vi "comm serial port list.vi"(8 "error in (no error)":errorcluster) -> (0 "error out":errorcluster, 3 "serial ports":string[](array[string]))   [LabVIEW 2013, in "lvserial.lvlib"]
doc: "Lists all serial ports and places them into a array."
uses:
  lvserial.lvlib
  lvserial.dll
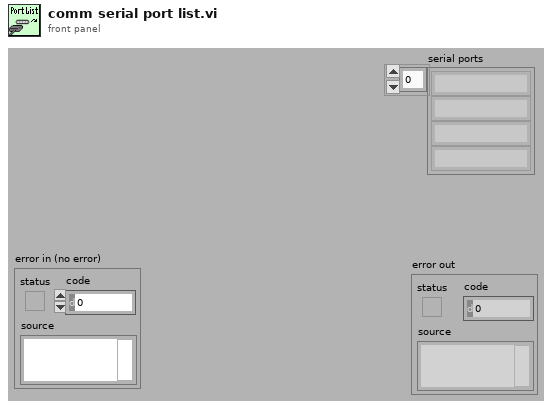
[diagram p1: front panel]
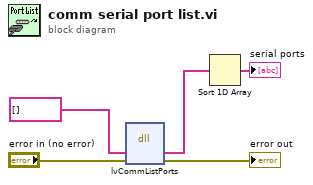
[diagram p0: block diagram]
diagram:
  n1 = dll-call lib="lvserial.dll" fn="lvCommListPorts"(string[] [], "error in (no error)"="error in (no error)") -> (w4:string[], "error in (no error)"=→"error out":errorcluster)  [unwired: 3 in, 3 out]
  n2 = Sort 1D Array(array=w4) -> (sorted array=→"serial ports":string[])
